vi "LagOneAutoCorr.vi"(8 "Doppler Params":T1={"Dopp Filter Order"=2, "Window length"=64, "Window Increment"=64, "Start f"=0.05, "lDoppler cutouff"=10.0, "FFT Length"=512, "SlowTime (Hz)"=100.0} {"Start f" format="%0.3f"; "SlowTime (Hz)" format="%0.1f"; "lDoppler cutouff" format="%0.3f"}, 10 "slow time":cdb[](array[numeric]), 11 "angular Scalar":dbl) -> (1 "FD,k":dbl, 2 "phase":dbl)   [LabVIEW 2022 SP3]
uses:
  DopplerParams.ctl
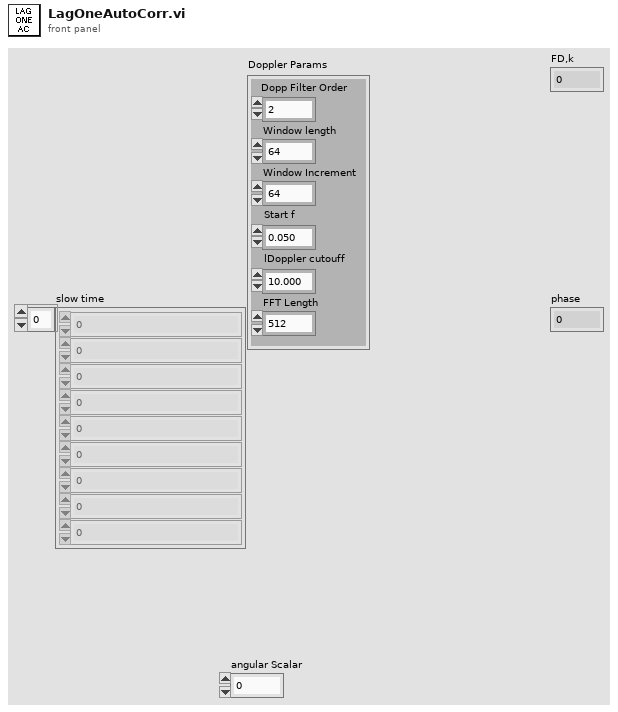
[diagram p1: front panel]
types:
  T1 = typedef "DopplerParams.ctl" = cluster{"Dopp Filter Order":i32, "Window length":i32, "Window Increment":i32, "Start f":dbl, "lDoppler cutouff":dbl, "FFT Length":i32, "SlowTime (Hz)":dbl}
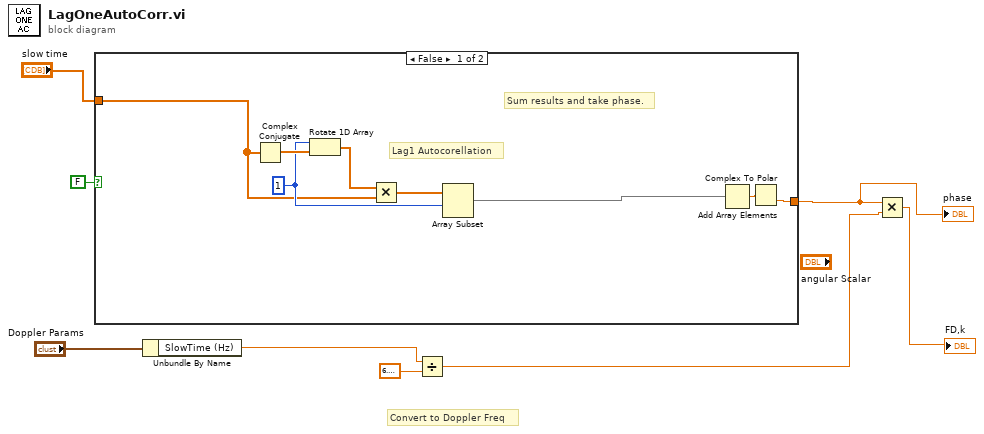
[diagram p0: block diagram]
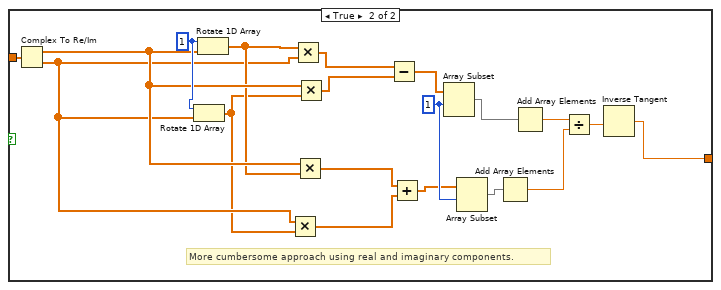
[diagram p2: hidden frame]
diagram:
  # "Convert to Doppler Freq"
  n1 = case shown="False" FALSE {
    tunnel: "slow time" -> [w10 w18]
    tunnel: [w14 w17] -> w2
    frame False {
      w11 = 1 ("n")
      # "Sum results and take phase."
      # "Lag1 Autocorellation"
      n2 = Complex Conjugate(1:w10) -> (0:w12:cdb[])
      n3 = Rotate 1D Array(1:w12, 2:w11) -> (0:w13:cdb[])
      n4 = Multiply(x=w13, y=w10) -> (x*y=w15:cdb[])
      n5 = Array Subset(array=w15, index=w11) -> (w9:cdb[])  [unwired: 1 in]
      n6 = Add Array Elements(numeric array=w9) -> (sum=w16:cdb)
      n7 = Complex To Polar(r * e^(i*theta)=w16) -> (theta=w14:dbl)  [unwired: 1 out]
    }
    frame True {
      w21 = 1 ("index")
      w35 = 1 ("n")
      # "More cumbersome approach using real and imaginary components."
      n8 = Complex To Re/Im(x + iy=w18) -> (x=w34:dbl[], y=w32:dbl[])
      n9 = Rotate 1D Array(1:w32, 2:w35) -> (0:w31:dbl[])
      n10 = Rotate 1D Array(1:w34, 2:w35) -> (0:w33:dbl[])
      n11 = Multiply(x=w32, y=w31) -> (x*y=w27:dbl[])
      n12 = Multiply(x=w33, y=w32) -> (x*y=w30:dbl[])
      n13 = Multiply(x=w34, y=w33) -> (x*y=w28:dbl[])
      n14 = Multiply(x=w34, y=w31) -> (x*y=w29:dbl[])
      n15 = Subtract(x=w30, y=w29) -> (x-y=w23:dbl[])
      n16 = Add(x=w28, y=w27) -> (x+y=w20:dbl[])
      n17 = Array Subset(array=w23, index=w21) -> (w19:dbl[])  [unwired: 1 in]
      n18 = Array Subset(array=w20, index=w21) -> (w22:dbl[])  [unwired: 1 in]
      n19 = Add Array Elements(numeric array=w22) -> (sum=w25:dbl)
      n20 = Add Array Elements(numeric array=w19) -> (sum=w26:dbl)
      n21 = Divide(x=w26, y=w25) -> (x/y=w24:dbl)
      n22 = Inverse Tangent(1:w24) -> (0:w17:dbl)
    }
  }
  "phase" <- w2
  n23 = Unbundle By Name("Doppler Params") -> ("SlowTime (Hz)"=w3:dbl)
  n24 = Divide(x=w3, y=6.283185307179586) -> (x/y=w5:dbl)
  n25 = Multiply(x=w2, y=w5) -> (x*y=→"FD,k":dbl)
